vi "F Dwf Analog IO Enable Info.vi"(8 "error in (no error)":errorcluster, 9 "pfStatus":i32, 10 "pfSet":i32, 11 "hdwf":i32) -> (0 "error out":errorcluster, 1 "pfStatus out":i32, 2 "pfSet out":i32, 3 "function return":i32)   [LabVIEW 2021, in "Olasdwf.lvlib"]
doc: "DWFAPI int FDwfAnalogIOEnableInfo(HDWF hdwf, int *pfSet, int *pfStatus);"
uses:
  Olasdwf.lvlib
  Windows/System32/dwf.dll
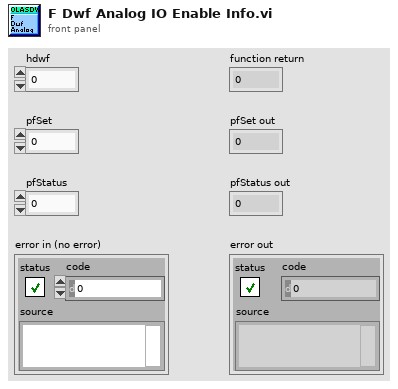
[diagram p1: front panel]
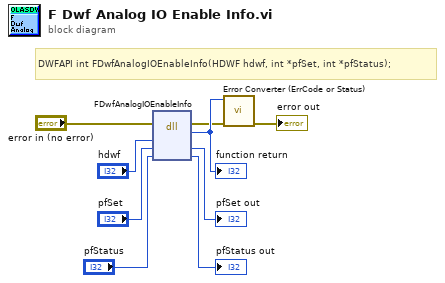
[diagram p0: block diagram]
diagram:
  # "DWFAPI int FDwfAnalogIOEnableInfo(HDWF hdwf, int *pfSet, int *pfStatus);"
  n1 = dll-call lib="/Windows/System32/dwf.*" fn="FDwfAnalogIOEnableInfo"(error in="error in (no error)", "hdwf"="hdwf", "pfSet"="pfSet", "pfStatus"="pfStatus") -> (error out=w2:errorcluster, w9:i32, "pfSet"=→"pfSet out":i32, "pfStatus"=→"pfStatus out":i32)  [unwired: 3 in, 1 out]
  "function return" <- w9
  n2 = call "Error Converter (ErrCode or Status).vi"("error in (no error)"=w2, "error code"=w9) -> ("error out"=→"error out":errorcluster)  [unwired: 9 in]
